vi "BufferedMax.vi"(7 "Buffer Size":i32, 11 "Signal":dbl) -> (3 "MaxValue":dbl)   [LabVIEW 2018]
doc: "Simple Low-Pass filter.\nAverages the last N samples."
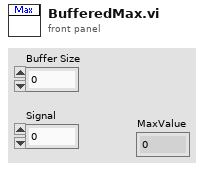
[diagram p1: front panel]
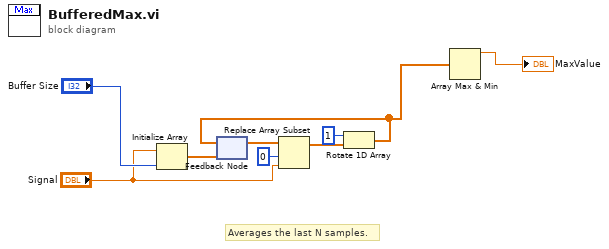
[diagram p0: block diagram]
diagram:
  # "Averages the last N samples."
  n1 = Initialize Array("Signal", "Buffer Size") -> (w5:dbl[])
  n2 = feedback #1(w5) -> (w7:dbl[])
  n3 = Replace Array Subset(array=w7, new element="Signal", index=0) -> (w8:dbl[])
  n4 = Rotate 1D Array(1:w8, 2:1 ("n")) -> (0:w2:dbl[])
  n5 = feedback-in #1(w2) -> ()
  n6 = Array Max & Min(array=w2) -> (max value=→"MaxValue":dbl)  [unwired: 3 out]
